vi "Tokenize Value Response.vi"(8 "error in (no error)":errorcluster, 10 "Input":string, 11 "Tovey 9150 in":refnum<class "Tovey 9150.lvclass">) -> (0 "error out":errorcluster, 2 "Tokens":string[](array[string]), 3 "Tovey 9150 out":refnum<class "Tovey 9150.lvclass">)   [LabVIEW 2015, in "Tovey 9150.lvclass"]
uses:
  Tovey 9150.lvclass
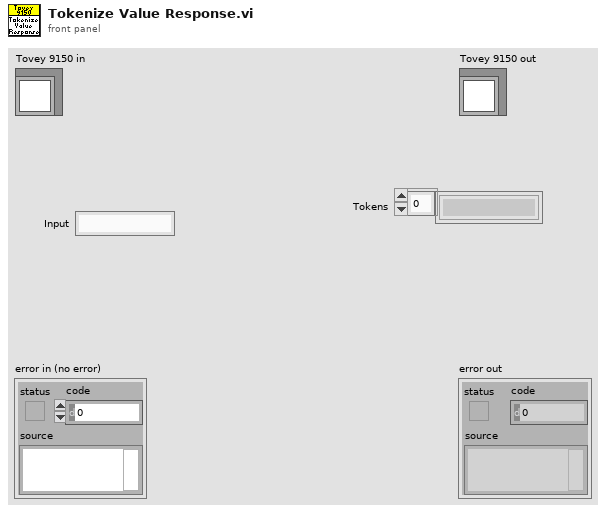
[diagram p1: front panel]
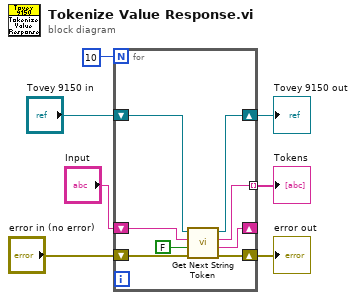
[diagram p0: block diagram]
diagram:
  n1 = for {
    N: 10 -> [_]
    shift-right: [w13] -> w6
    shift-left: "Tovey 9150 in" -> [w14]
    shift-right: [w12] -> _
    shift-left: "Input" -> [w15]
    tunnel: [w11] -> w2 mode=indexing
    shift-right: [w9] -> w4
    shift-left: "error in (no error)" -> [w10]
    n2 = call "Get Next String Token.vi"("error in (no error)"=w10, "Final"=FALSE, "inputString"=w15, "TEI9150 in"=w14) -> ("error out"=w9:errorcluster, "remainingString"=w12:string, "extractedSegment"=w11:string, "TEI9150 out"=w13:refnum<class "Tovey 9150.lvclass">)  [unwired: 4 in]
  }
  "error out" <- w4
  "Tovey 9150 out" <- w6
  "Tokens" <- w2
